vi "2HP_Create datalog header string.vi"() -> (0 "Datalog header string":string)   [LabVIEW 2018]
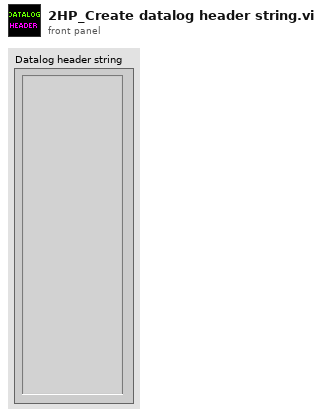
[diagram p1: front panel]
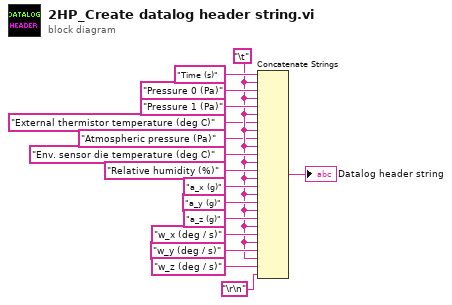
[diagram p0: block diagram]
diagram:
  w3 = "\t"
  n1 = Concatenate Strings("Time (s)", w3, "Pressure 0 (Pa)", w3, "Pressure 1 (Pa)", w3, "External thermistor temperature (deg C)", w3, "Atmospheric pressure (Pa)", w3, "Env. sensor die temperature (deg C)", w3, "Relative humidity (%)", w3, "a_x (g)", w3, "a_y (g)", w3, "a_z (g)", w3, "w_x (deg / s)", w3, "w_y (deg / s)", w3, "w_z (deg / s)", "\r\n") -> (→"Datalog header string":string)
